vi "超标留样不超标排空.vi"(8 "error in (no error)":errorcluster) -> (0 "error out":errorcluster)   [LabVIEW 2016, in "超标留样集成.lvlib" / "ESTD1200.lvlib"]
uses:
  ESTD1200.lvlib
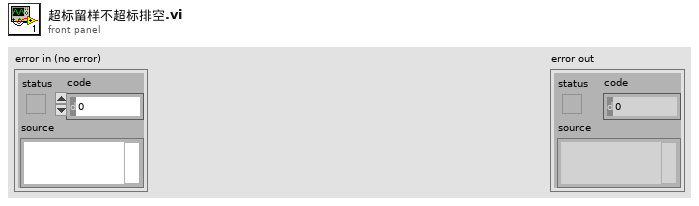
[diagram p1: front panel]
types:
  T1 = enum16{"open", "read", "write", "write single", "close"}
  T2 = cluster{"STEP":enum16{"open", "read", "write", "write single", "close"}, "starting address":u16, "value":u16}
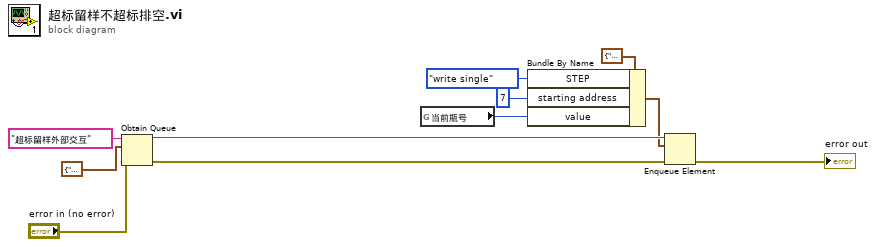
[diagram p0: block diagram]
diagram:
  n1 = Obtain Queue(name (unnamed)="超标留样外部交互" ("名称（未命名）"), element data type=T2 {"STEP"=enum."write single", "starting address"=0, "value"=0}, error in (no error)="error in (no error)") -> (queue out=w6:refnum<queue>, error out=w4:errorcluster)  [unwired: 2 in, 1 out]
  n2 = global read "超标留样全局.vi" "当前瓶号"() -> (w2:u16)
  n3 = Bundle By Name(cluster=T2 {"STEP"=enum."open", "starting address"=0, "value"=0} ("元素"), "STEP"=T1."write single", "starting address"=7 ("索引"), "value"=w2) -> (w5:T2)
  n4 = Enqueue Element(queue=w6, element=w5, error in (no error)=w4) -> (error out=→"error out":errorcluster)  [unwired: 1 in, 2 out]
